vi "ConversioneDati.vi"(4 "Stato Conversione":enum16{"CONVERTI_IN", "CONVERTI_OUT"}(ring), 10 "Data":dbl, 11 "Impostazioni Conversione":string[](array[string])) -> (3 "Dato Convertito":dbl)   [LabVIEW 2019]
uses:
  <vilib>/gmath/NI_Gmath.lvlib
panel:
  out "element":dbl
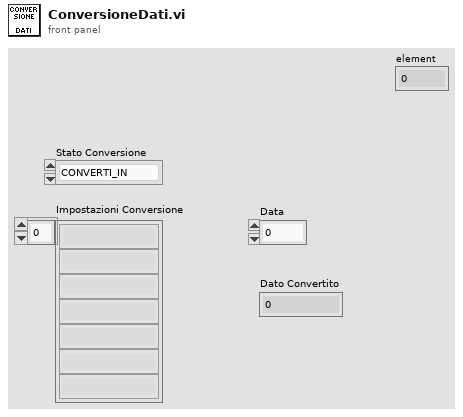
[diagram p1: front panel]
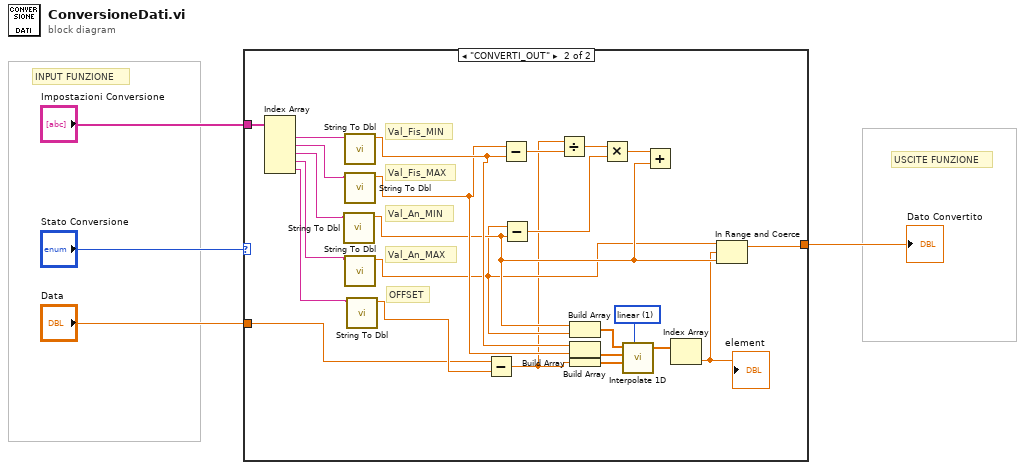
[diagram p0: block diagram]
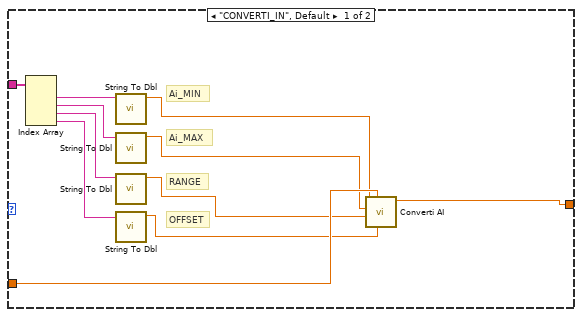
[diagram p2: hidden frame]
diagram:
  # "USCITE FUNZIONE"
  # "INPUT FUNZIONE"
  n1 = case shown="\"CONVERTI_OUT\"" "Stato Conversione" {
    tunnel: "Impostazioni Conversione" -> [w15 w39]
    tunnel: [w14 w38] -> w3
    tunnel: "Data" -> [w13 w26]
    frame "CONVERTI_IN", Default {
      # "OFFSET"
      # "RANGE"
      # "Ai_MAX"
      # "Ai_MIN"
      n2 = Index Array(array=w15) -> (element #1=w12:string, element #2=w10:string, element #3=w8:string, element #4=w6:string)  [unwired: 4 in]
      n3 = call "String To Dbl.vi"("String"=w12) -> ("Numeric"=w11:dbl)  [unwired: 10 in]
      n4 = call "String To Dbl.vi"("String"=w10) -> ("Numeric"=w9:dbl)  [unwired: 10 in]
      n5 = call "String To Dbl.vi"("String"=w8) -> ("Numeric"=w7:dbl)  [unwired: 10 in]
      n6 = call "String To Dbl.vi"("String"=w6) -> ("Numeric"=w5:dbl)  [unwired: 10 in]
      n7 = call "Converti AI.vi"("Offset"=w5, "Dato"=w13, "Range"=w7, "Ai_MAX"=w9, "AI min"=w11) -> ("Dato convertito"=w14:dbl)  [unwired: 6 in]
    }
    frame "CONVERTI_OUT" {
      w19 = 1 items=["nearest", "linear", "spline", "cubic Hermite", "Lagrange"] ("method")
      # "OFFSET"
      # "Val_An_MAX"
      # "Val_An_MIN"
      # "Val_Fis_MAX"
      # "Val_Fis_MIN"
      n8 = Index Array(array=w39) -> (element #1=w33:string, element #2=w32:string, element #3=w31:string, element #4=w30:string, element #5=w29:string)  [unwired: 5 in]
      n9 = call "String To Dbl.vi"("String"=w31) -> ("Numeric"=w21:dbl)  [unwired: 10 in]
      n10 = call "String To Dbl.vi"("String"=w33) -> ("Numeric"=w23:dbl)  [unwired: 10 in]
      n11 = call "String To Dbl.vi"("String"=w32) -> ("Numeric"=w22:dbl)  [unwired: 10 in]
      n12 = call "String To Dbl.vi"("String"=w30) -> ("Numeric"=w20:dbl)  [unwired: 10 in]
      n13 = call "String To Dbl.vi"("String"=w29) -> ("Numeric"=w28:dbl)  [unwired: 10 in]
      n14 = Subtract(x=w26, y=w28) -> (x-y=w17:dbl)
      n15 = Subtract(x=w22, y=w23) -> (x-y=w37:dbl)
      n16 = Subtract(x=w20, y=w21) -> (x-y=w34:dbl)
      n17 = Divide(x=w17, y=w37) -> (x/y=w36:dbl)
      n18 = Build Array(w21, w20) -> (w24:dbl[])
      n19 = Build Array(w23, w22) -> (w25:dbl[])
      n20 = Build Array(w17) -> (w27:dbl[])
      n21 = Multiply(x=w36, y=w34) -> (x*y=w35:dbl)
      n22 = call <vilib>:"Interpolate 1D.vi"("method"=w19, "xi"=w27, "X"=w25, "Y"=w24) -> ("yi"=w18:dbl[])  [unwired: 5 in, 2 out]
      n23 = Add(x=w35, y=w21) -> ()  [unwired: 1 out]
      n24 = Index Array(array=w18) -> (element=w16:dbl)  [unwired: 1 in]
      "element" <- w16
      n25 = In Range and Coerce(upper limit=w20, x=w16, lower limit=w21) -> (coerced(x)=w38:dbl)  [unwired: 1 out]
    }
  }
  "Dato Convertito" <- w3
